vi "Servo Pulse Gen..vi"() -> ()   [LabVIEW 2015]
uses:
  Slide Servo.ctl
  Galobal variable_TI.vi
  Project Setup/Globle Variable/GR_Servo.vi
panel:
  out "Enum":T1
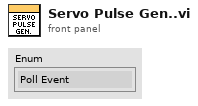
[diagram p1: front panel]
types:
  T1 = typedef "Slide Servo.ctl" = enum16{"Poll Event", "Servo CMD", "Slide Servo Home ", "Exit"}
  T2 = cluster{"Emergency_1":bool, "Reset_2":bool, "Home _3":bool, "Air Pressure_4":bool, "Safety Sensor_5":bool, "Safety Sensor_6":bool, "Slide Servo Home RS 26":bool, "LVDT UP RS":bool, "Servo Fault 27":bool, "Pressing UP RS 31":bool, "40 Deg. Down Fixture Rs":bool}
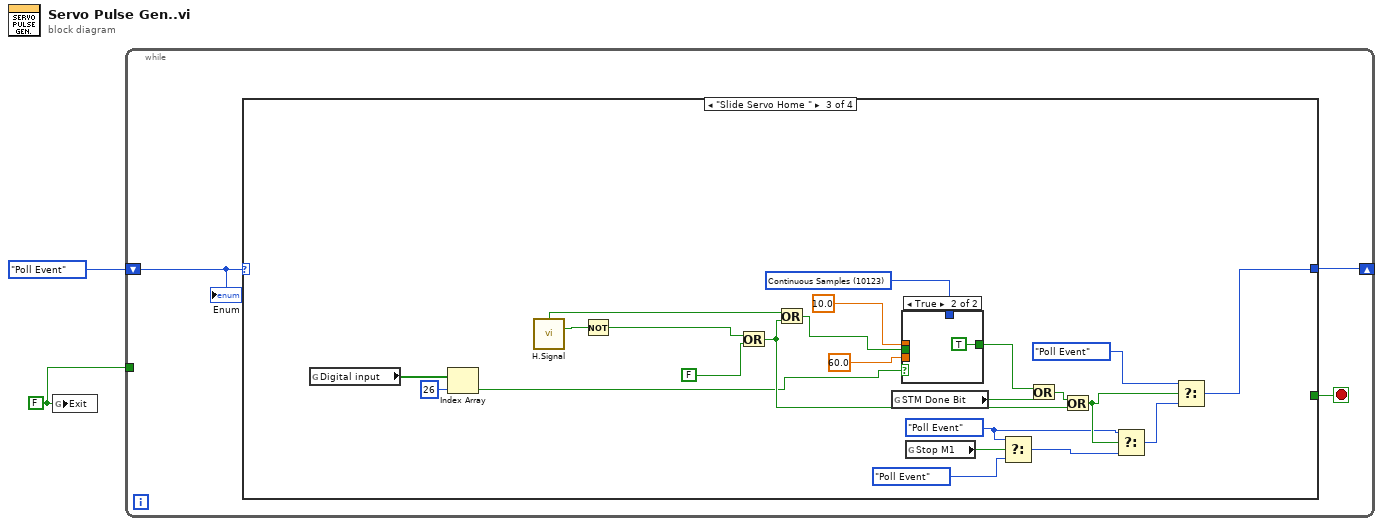
[diagram p0: block diagram]
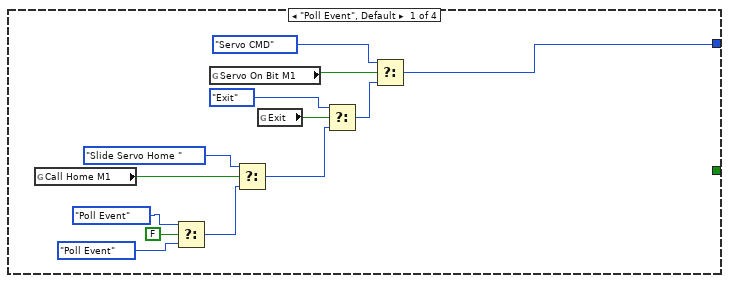
[diagram p2: hidden frame]
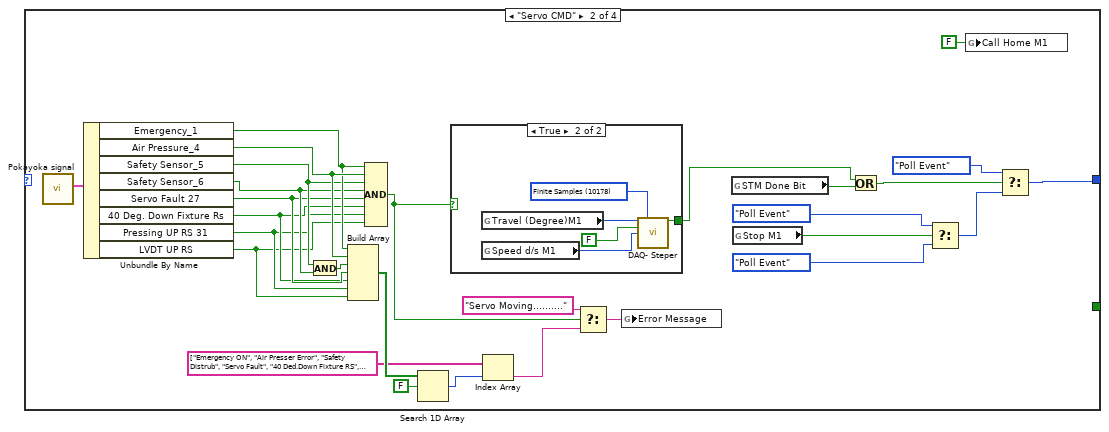
[diagram p3: hidden frame]
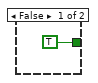
[diagram p4: hidden frame]
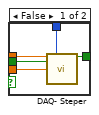
[diagram p5: hidden frame]
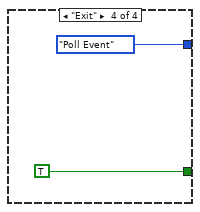
[diagram p6: hidden frame]
diagram:
  w1 = FALSE ("Exit")
  n1 = global write "Galobal variable_TI.vi" "Exit"(w1) -> ()
  n2 = while {
    shift-right: [w4] -> _
    shift-left: Slide_Servo."Poll Event" ("Enum") -> [w5]
    tunnel: w1 -> [_]
    stop <- w3 stop-if-true
    n3 = case shown="\"Slide Servo Home \"" w5 {
      tunnel: [w13 w42 w64 Slide_Servo."Poll Event" ("Enum")] -> w4
      tunnel: [_ _ _ TRUE] -> w3
      frame "Poll Event", Default {
        n4 = global read "Galobal variable_TI.vi" "Call Home M1"() -> (w11:bool)
        n5 = Select(t=Slide_Servo."Poll Event" ("Enum"), s=FALSE, f=Slide_Servo."Poll Event" ("Enum")) -> (s? t:f=w8:T1)
        n6 = global read "GR_Servo.vi" "Servo On Bit M1"() -> (w16:bool)
        n7 = Select(t=Slide_Servo."Slide Servo Home " ("Enum"), s=w11, f=w8) -> (s? t:f=w10:T1)
        n8 = global read "Galobal variable_TI.vi" "Exit"() -> (w17:bool)
        n9 = Select(t=Slide_Servo."Exit" ("Enum"), s=w17, f=w10) -> (s? t:f=w18:T1)
        n10 = Select(t=Slide_Servo."Servo CMD" ("Enum"), s=w16, f=w18) -> (s? t:f=w13:T1)
      }
      frame "Servo CMD" {
        n11 = call "Pokayoka signal.vi"() -> ("output cluster"=w34:T2)  [unwired: 10 in, 1 out]
        n12 = Unbundle By Name(w34) -> ("Emergency_1"=w31:bool, "Air Pressure_4"=w32:bool, "Safety Sensor_5"=w30:bool, "Safety Sensor_6"=w29:bool, "Servo Fault 27"=w27:bool, "40 Deg. Down Fixture Rs"=w26:bool, "Pressing UP RS 31"=w25:bool, "LVDT UP RS"=w24:bool)
        n13 = And(x=w30, y=w29) -> (x .and. y?=w28:bool)
        n14 = Build Array(w31, w32, w28, w27, w26, w25, w24) -> (w23:bool[])
        n15 = Compound Arithmetic op=AND(w31, w32, w30, w29, w27, w26, w25, w24) -> (w33:bool)
        n16 = Search 1D Array(1D array=w23, element=FALSE) -> (index of element=w21:i32)  [unwired: 1 in]
        n17 = case shown="True" w33 {
          tunnel: [TRUE ("Task Done Bit") w50] -> w46
          frame False {
          }
          frame True {
            w48 = 10178 items=["Finite Samples"=10178, "Continuous Samples"=10123, "Hardware Timed Single Point"=12522] ("Mode")
            n18 = global read "GR_Servo.vi" "Travel (Degree)M1"() -> (w51:i32)
            n19 = global read "GR_Servo.vi" "Speed d/s M1"() -> (w52:i32)
            n20 = call "DAQ- Steper.vi"("Travel (Degree)"=w51, "Mode"=w48, "Home Condition"=FALSE, "Speed d/s"=w52) -> ("Task Done Bit"=w50:bool)  [unwired: 10 in, 1 out]
          }
        }
        n21 = Index Array(array=string[] ["Emergency ON", "Air Presser Error", "Safety Distrub", "Servo Fault", "40 Ded.Down Fixture RS", "Pressing UP RS", "LVDT UP RS"], index=w21) -> (element=w19:string)
        n22 = Select(t="Servo Moving..........", s=w33, f=w19) -> (s? t:f=w35:string)
        n23 = global write "GR_Servo.vi" "Error Message"(w35) -> ()
        n24 = global read "Galobal variable_TI.vi" "STM Done Bit"() -> (w45:bool)
        n25 = global read "Galobal variable_TI.vi" "Stop M1"() -> (w41:bool)
        n26 = Or(x=w46, y=w45) -> (x .or. y?=w44:bool)
        n27 = Select(t=Slide_Servo."Poll Event" ("Enum"), s=w41, f=Slide_Servo."Poll Event" ("Enum")) -> (s? t:f=w38:T1)
        n28 = global write "Galobal variable_TI.vi" "Call Home M1"(FALSE ("Call Home M1")) -> ()
        n29 = Select(t=Slide_Servo."Poll Event" ("Enum"), s=w44, f=w38) -> (s? t:f=w42:T1)
      }
      frame "Slide Servo Home " {
        w63 = 10123 items=["Finite Samples"=10178, "Continuous Samples"=10123, "Hardware Timed Single Point"=12522] ("Mode")
        w66 = Slide_Servo."Poll Event" ("Enum")
        n30 = global read "Galobal variable_TI.vi" "Digital input"() -> (w55:bool[])
        n31 = Index Array(array=w55, index=26) -> (element=w53:bool)
        n32 = call "H.Signal.vi"() -> ("element"=w57:bool, "HI Bit Auto"=w60:bool)  [unwired: 10 in, 4 out]
        n33 = Not(x=w60) -> (.not. x?=w59:bool)
        n34 = Or(x=w59, y=FALSE) -> (x .or. y?=w58:bool)
        n35 = Or(x=w57, y=w58) -> (x .or. y?=w56:bool)
        n36 = global read "Galobal variable_TI.vi" "STM Done Bit"() -> (w74:bool)
        n37 = case shown="True" w53 {
          tunnel: [w80 TRUE ("Task Done Bit")] -> w75
          tunnel: w63 -> [w79 _]
          tunnel: 10.0 ("Travel (Degree)") -> [w78 _]
          tunnel: 60.0 ("Speed d/s") -> [w77 _]
          tunnel: w56 -> [w76 _]
          frame False {
            n38 = call "DAQ- Steper.vi"("Travel (Degree)"=w78, "Mode"=w79, "Home Condition"=w76, "Speed d/s"=w77) -> ("Task Done Bit"=w80:bool)  [unwired: 10 in, 1 out]
          }
          frame True {
          }
        }
        n39 = global read "Galobal variable_TI.vi" "Stop M1"() -> (w70:bool)
        n40 = Select(t=w66, s=w70, f=Slide_Servo."Poll Event" ("Enum")) -> (s? t:f=w67:T1)
        n41 = Or(x=w75, y=w74) -> (x .or. y?=w71:bool)
        n42 = Or(x=w71, y=w58) -> (x .or. y?=w68:bool)
        n43 = Select(t=w66, s=w68, f=w67) -> (s? t:f=w65:T1)
        n44 = Select(t=Slide_Servo."Poll Event" ("Enum"), s=w68, f=w65) -> (s? t:f=w64:T1)
      }
      frame "Exit" {
      }
    }
    "Enum" <- w5
  }
